vi "FTW-JSON-LexicalScan-Number.vi"(0 "JSON String":T1, 11 "error in":errorcluster) -> (4 "JSON String Out":T1, 8 "Number":variant, 15 "error out":errorcluster)   [LabVIEW 2015]
uses:
  FTW-JSON-LexicalScan.ctl
panel:
  # "Inputs"
  # "Outputs"
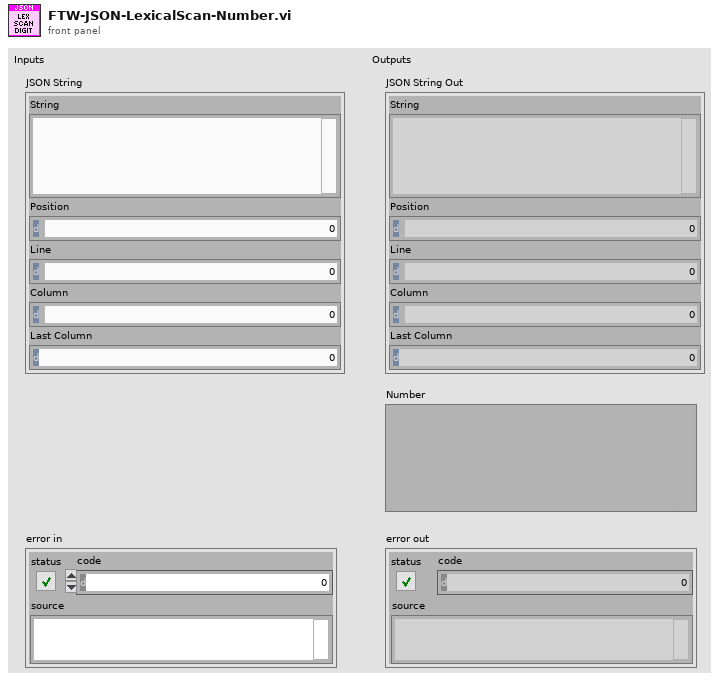
[diagram p1: front panel]
types:
  T1 = typedef "FTW-JSON-LexicalScan.ctl" = cluster{"String":string, "Position":i32, "Line":i32, "Column":i32, "Last Column":i32}
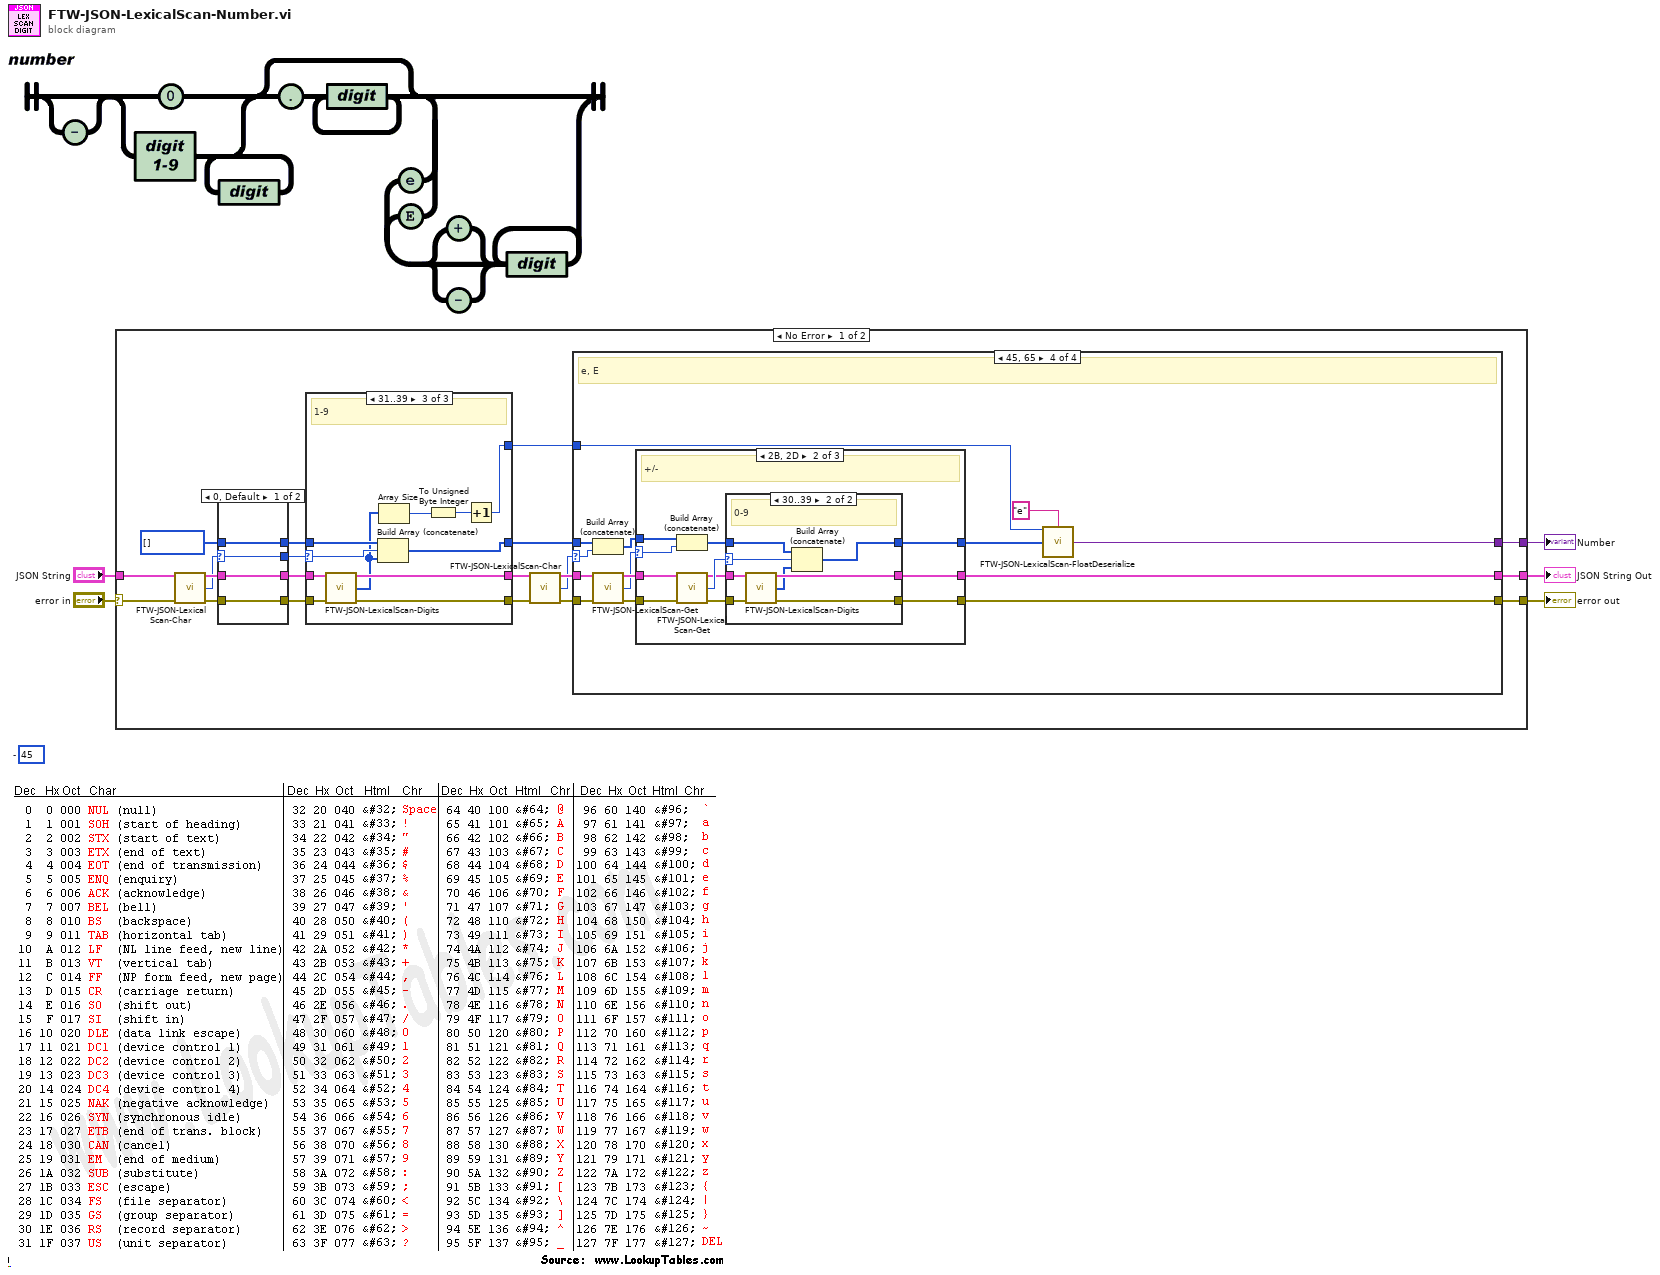
[diagram p0: block diagram]
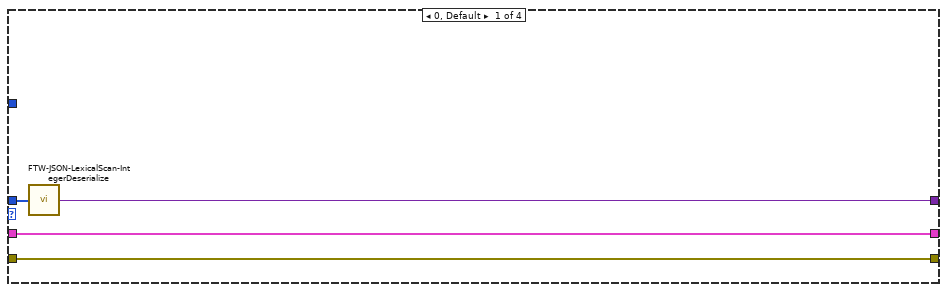
[diagram p2: hidden frame]
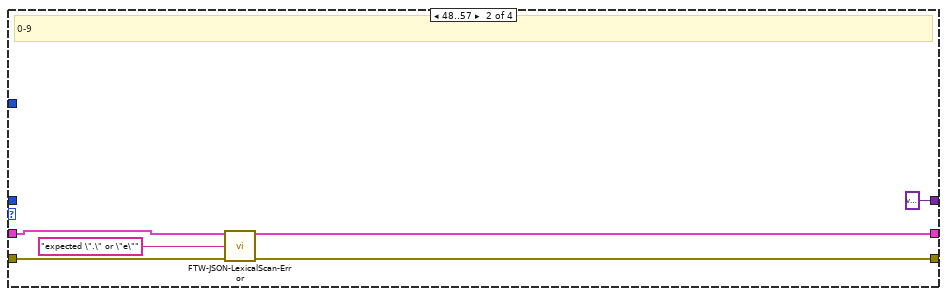
[diagram p3: hidden frame]
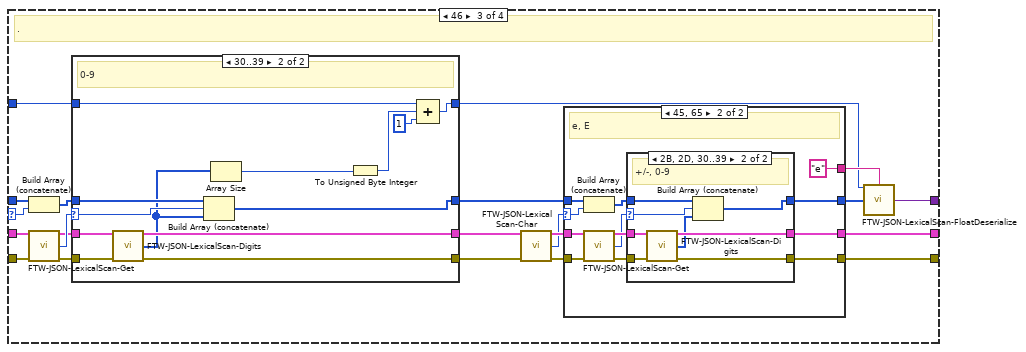
[diagram p4: hidden frame]
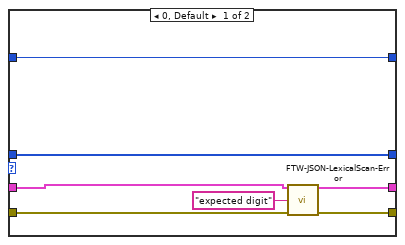
[diagram p5: hidden frame]
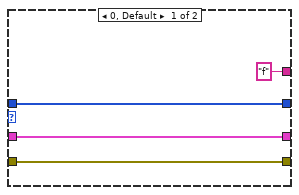
[diagram p6: hidden frame]
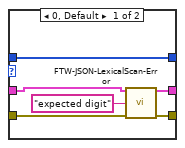
[diagram p7: hidden frame]
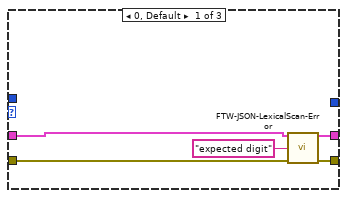
[diagram p8: hidden frame]
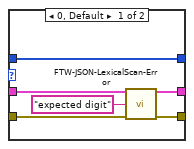
[diagram p9: hidden frame]
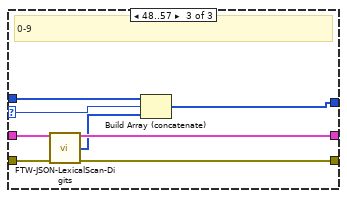
[diagram p10: hidden frame]
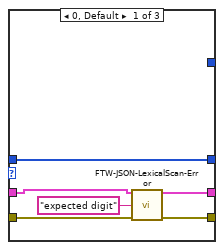
[diagram p11: hidden frame]
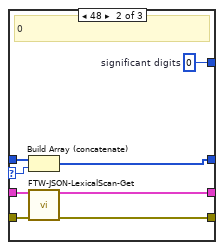
[diagram p12: hidden frame]
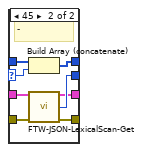
[diagram p13: hidden frame]
diagram:
  (unwired) u8 45  # -
  n1 = case shown="No Error" "error in" {
    selector: "error in" -> [w24 w197]
    tunnel: "JSON String" -> [w25 w196]
    tunnel: [w7 w197] -> w5
    tunnel: [w8 w196] -> w4
    tunnel: [w15 _] -> w1
    frame No Error {
      n2 = call "FTW-JSON-LexicalScan-Char.vi"("JSON String"=w25, "error in"=w24) -> ("JSON String Out"=w14:T1, "Char"=w9:u8, "error out"=w13:errorcluster)  [unwired: 11 in]
      n3 = case shown="0, Default" w9 {
        selector: w9 -> [w184 w188]
        tunnel: u8[] [] -> [w187 w195]
        tunnel: [w187 w194] -> w22
        tunnel: w14 -> [w186 w193]
        tunnel: w13 -> [w185 w192]
        tunnel: [w185 w191] -> w12
        tunnel: [w184 w190] -> w11
        tunnel: [w186 w189] -> w10
        frame 0, Default {
        }
        frame 45 {
          # "-"
          n4 = Build Array (concatenate)(w195, w188) -> (w194:u8[])
          n5 = call "FTW-JSON-LexicalScan-Get.vi"("JSON String"=w193, "error in"=w192) -> ("JSON String Out"=w189:T1, "Char"=w190:u8, "error out"=w191:errorcluster)  [unwired: 11 in]
        }
      }
      n6 = case shown="31..39" w11 {
        selector: w11 -> [_ w170 w182]
        tunnel: w12 -> [w164 w172 w180]
        tunnel: w10 -> [w163 w167 w179]
        tunnel: [w160 w166 w177] -> w18
        tunnel: [w159 w168 w178] -> w21
        tunnel: w22 -> [w161 w171 w183]
        tunnel: [w161 w169 w181] -> w20
        tunnel: [_ w165 w174] -> w6
        frame 0, Default {
          n7 = call "FTW-JSON-LexicalScan-Error.vi"("JSON String"=w163, "Error String"="expected digit", "error in"=w164) -> ("JSON String Out"=w160:T1, "error out"=w159:errorcluster)  [unwired: 11 in]
        }
        frame 48 {
          w165 = u8 0  # significant digits
          # "0"
          n8 = Build Array (concatenate)(w171, w170) -> (w169:u8[])
          n9 = call "FTW-JSON-LexicalScan-Get.vi"("JSON String"=w167, "error in"=w172) -> ("JSON String Out"=w166:T1, "error out"=w168:errorcluster)  [unwired: 11 in, 1 out]
        }
        frame 49..57 {
          # "1-9"
          n10 = call "FTW-JSON-LexicalScan-Digits.vi"("JSON String"=w179, "error in"=w180) -> ("JSON String Out"=w177:T1, "Digits"=w176:u8[], "error out"=w178:errorcluster)  [unwired: 11 in]
          n11 = Build Array (concatenate)(w183, w182, w176) -> (w181:u8[])
          n12 = Array Size(array=w176) -> (size(s)=w175:i32)
          n13 = To Unsigned Byte Integer(number=w175) -> (unsigned 8bit integer=w173:u8)
          n14 = Increment(x=w173) -> (x+1=w174:u8)
        }
      }
      n15 = call "FTW-JSON-LexicalScan-Char.vi"("JSON String"=w18, "error in"=w21) -> ("JSON String Out"=w17:T1, "Char"=w16:u8, "error out"=w19:errorcluster)  [unwired: 11 in]
      n16 = case shown="45, 65" w16 {
        selector: w16 -> [_ _ w55 w119]
        tunnel: w19 -> [w29 w33 w46 w118]
        tunnel: w17 -> [w28 w34 w45 w116]
        tunnel: [w28 w32 w51 w112] -> w8
        tunnel: [w29 w31 w50 w111] -> w7
        tunnel: w20 -> [w27 _ w56 w120]
        tunnel: [w26 variant ("Variant") w37 w107] -> w15
        tunnel: w6 -> [_ _ w40 w108]
        frame 0, Default {
          n17 = call "FTW-JSON-LexicalScan-IntegerDeserialize.vi"("Byte Array"=w27) -> ("Variant"=w26:variant)  [unwired: 14 in]
        }
        frame 48..57 {
          # "0-9"
          n18 = call "FTW-JSON-LexicalScan-Error.vi"("JSON String"=w34, "Error String"="expected \".\" or \"e\"", "error in"=w33) -> ("JSON String Out"=w32:T1, "error out"=w31:errorcluster)  [unwired: 11 in]
        }
        frame 46 {
          # "."
          n19 = Build Array (concatenate)(w56, w55) -> (w42:u8[])
          n20 = call "FTW-JSON-LexicalScan-Get.vi"("JSON String"=w45, "error in"=w46) -> ("JSON String Out"=w48:T1, "Char"=w49:u8, "error out"=w47:errorcluster)  [unwired: 11 in]
          n21 = case shown="30..39" w49 {
            selector: w49 -> [_ w75]
            tunnel: w47 -> [w63 w72]
            tunnel: w48 -> [w62 w73]
            tunnel: [w59 w71] -> w43
            tunnel: [w58 w70] -> w44
            tunnel: w42 -> [w60 w76]
            tunnel: [w60 w74] -> w41
            tunnel: w40 -> [w57 w69]
            tunnel: [w57 w65] -> w36
            frame 0, Default {
              n22 = call "FTW-JSON-LexicalScan-Error.vi"("JSON String"=w62, "Error String"="expected digit", "error in"=w63) -> ("JSON String Out"=w59:T1, "error out"=w58:errorcluster)  [unwired: 11 in]
            }
            frame 48..57 {
              # "0-9"
              n23 = call "FTW-JSON-LexicalScan-Digits.vi"("JSON String"=w73, "error in"=w72) -> ("JSON String Out"=w71:T1, "Digits"=w68:u8[], "error out"=w70:errorcluster)  [unwired: 11 in]
              n24 = Build Array (concatenate)(w76, w75, w68) -> (w74:u8[])
              n25 = Array Size(array=w68) -> (size(s)=w67:i32)
              n26 = To Unsigned Byte Integer(number=w67) -> (unsigned 8bit integer=w64:u8)
              n27 = Compound Arithmetic op=ADD(w69, w64, u8 1 ("value")) -> (w65:u8)
            }
          }
          n28 = call "FTW-JSON-LexicalScan-Char.vi"("JSON String"=w43, "error in"=w44) -> ("JSON String Out"=w53:T1, "Char"=w52:u8, "error out"=w54:errorcluster)  [unwired: 11 in]
          n29 = case shown="45, 65" w52 {
            selector: w52 -> [_ w91]
            tunnel: w54 -> [w80 w90]
            tunnel: w53 -> [w79 w88]
            tunnel: [w79 w84] -> w51
            tunnel: [w80 w83] -> w50
            tunnel: w41 -> [w78 w92]
            tunnel: [w78 w81] -> w39
            tunnel: ["f" ("format string") "e" ("format string")] -> w38
            frame 0, Default {
            }
            frame 69, 101 {
              # "e, E"
              n30 = Build Array (concatenate)(w92, w91) -> (w85:u8[])
              n31 = call "FTW-JSON-LexicalScan-Get.vi"("JSON String"=w88, "error in"=w90) -> ("JSON String Out"=w87:T1, "Char"=w86:u8, "error out"=w89:errorcluster)  [unwired: 11 in]
              n32 = case shown="2B, 2D, 30..39" w86 {
                selector: w86 -> [_ w105]
                tunnel: w89 -> [w98 w102]
                tunnel: w87 -> [w97 w103]
                tunnel: [w94 w101] -> w84
                tunnel: [w93 w100] -> w83
                tunnel: w85 -> [w95 w106]
                tunnel: [w95 w104] -> w81
                frame 0, Default {
                  n33 = call "FTW-JSON-LexicalScan-Error.vi"("JSON String"=w97, "Error String"="expected digit", "error in"=w98) -> ("JSON String Out"=w94:T1, "error out"=w93:errorcluster)  [unwired: 11 in]
                }
                frame 43, 45, 48..57 {
                  # "+/-, 0-9"
                  n34 = call "FTW-JSON-LexicalScan-Digits.vi"("JSON String"=w103, "error in"=w102) -> ("JSON String Out"=w101:T1, "Digits"=w99:u8[], "error out"=w100:errorcluster)  [unwired: 11 in]
                  n35 = Build Array (concatenate)(w106, w105, w99) -> (w104:u8[])
                }
              }
            }
          }
          n36 = call "FTW-JSON-LexicalScan-FloatDeserialize.vi"("Significant Digits"=w36, "Format"=w38, "Byte Array"=w39) -> ("Variant"=w37:variant)  [unwired: 12 in]
        }
        frame 69, 101 {
          # "e, E"
          n37 = Build Array (concatenate)(w120, w119) -> (w113:u8[])
          n38 = call "FTW-JSON-LexicalScan-Get.vi"("JSON String"=w116, "error in"=w118) -> ("JSON String Out"=w115:T1, "Char"=w114:u8, "error out"=w117:errorcluster)  [unwired: 11 in]
          n39 = case shown="2B, 2D" w114 {
            selector: w114 -> [_ w127 w157]
            tunnel: w117 -> [w125 w131 w156]
            tunnel: w115 -> [w124 w130 w155]
            tunnel: [w122 w128 w153] -> w112
            tunnel: [w121 w129 w154] -> w111
            tunnel: w113 -> [_ w136 w158]
            tunnel: [_ w126 w151] -> w109
            frame 0, Default {
              n40 = call "FTW-JSON-LexicalScan-Error.vi"("JSON String"=w124, "Error String"="expected digit", "error in"=w125) -> ("JSON String Out"=w122:T1, "error out"=w121:errorcluster)  [unwired: 11 in]
            }
            frame 43, 45 {
              # "+/-"
              n41 = Build Array (concatenate)(w136, w127) -> (w132:u8[])
              n42 = call "FTW-JSON-LexicalScan-Get.vi"("JSON String"=w130, "error in"=w131) -> ("JSON String Out"=w134:T1, "Char"=w135:u8, "error out"=w133:errorcluster)  [unwired: 11 in]
              n43 = case shown="30..39" w135 {
                selector: w135 -> [_ w149]
                tunnel: w133 -> [w142 w146]
                tunnel: w134 -> [w141 w147]
                tunnel: [w138 w145] -> w128
                tunnel: [w137 w144] -> w129
                tunnel: w132 -> [w139 w150]
                tunnel: [w139 w148] -> w126
                frame 0, Default {
                  n44 = call "FTW-JSON-LexicalScan-Error.vi"("JSON String"=w141, "Error String"="expected digit", "error in"=w142) -> ("JSON String Out"=w138:T1, "error out"=w137:errorcluster)  [unwired: 11 in]
                }
                frame 48..57 {
                  # "0-9"
                  n45 = call "FTW-JSON-LexicalScan-Digits.vi"("JSON String"=w147, "error in"=w146) -> ("JSON String Out"=w145:T1, "Digits"=w143:u8[], "error out"=w144:errorcluster)  [unwired: 11 in]
                  n46 = Build Array (concatenate)(w150, w149, w143) -> (w148:u8[])
                }
              }
            }
            frame 48..57 {
              # "0-9"
              n47 = call "FTW-JSON-LexicalScan-Digits.vi"("JSON String"=w155, "error in"=w156) -> ("JSON String Out"=w153:T1, "Digits"=w152:u8[], "error out"=w154:errorcluster)  [unwired: 11 in]
              n48 = Build Array (concatenate)(w158, w157, w152) -> (w151:u8[])
            }
          }
          n49 = call "FTW-JSON-LexicalScan-FloatDeserialize.vi"("Significant Digits"=w108, "Format"="e" ("format string"), "Byte Array"=w109) -> ("Variant"=w107:variant)  [unwired: 12 in]
        }
      }
    }
    frame Error {
    }
  }
  "Number" <- w1
  "error out" <- w5
  "JSON String Out" <- w4
